vi "poly_notify_by_name_multi.vi"(8 "error in":errorcluster caption="Error in (no error)", 9 "notifier names":string[](array[string]), 10 "name of caller in":string) -> (0 "error out":errorcluster, 1 "notifier refs out":refnum<vi>[](array[refnum]), 4 "notified?":bool[](array[boolean]))   [LabVIEW 2015]
uses:
  ref_tools/polys/poly_control_ref_from_name_caller_multi.vi
  ref_tools/ref_tools_eco.vi
  ref_tools/polys/poly_ref_tools_eco_plus.vi
  error_tools/error_handler.vi
  ref_tools/polys/poly_control_ref_from_name_multi.vi
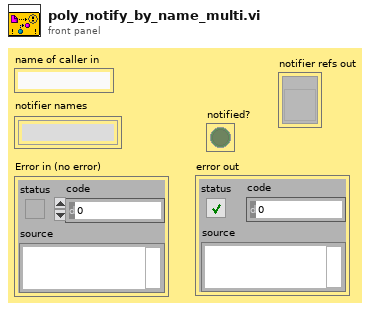
[diagram p1: front panel]
types:
  T1 = typedef "boolean_notifier.ctl" = refnum<notifier>
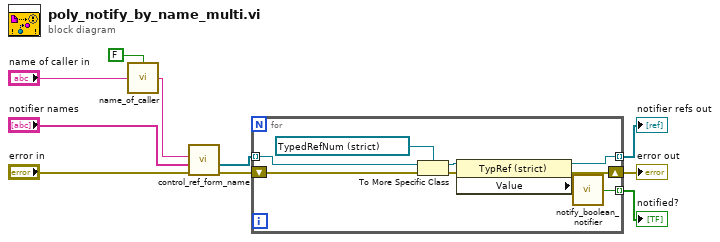
[diagram p0: block diagram]
diagram:
  n1 = call "name_of_caller.vi"("is in inlined vi? (F)"=FALSE, "name of caller in"="name of caller in") -> ("name of caller out"=w6:string)  [unwired: 2 in]
  n2 = call-poly "control_ref_form_name.vi"("error in"="error in", "control names"="notifier names", "name of caller in (your caller)"=w6) -> ("error out"=w8:errorcluster, "control refs"=w10:refnum<vi>[])  [unwired: 6 in, 1 out]
  n3 = for {
    tunnel: w10 -> [w19] mode=indexing
    tunnel: [w12] -> w1 mode=indexing
    tunnel: [w11] -> w2 mode=indexing
    shift-right: [w13] -> w7
    shift-left: w8 -> [w15]
    n4 = To More Specific Class(target class=refnum<vi> refnum ("notifier"), reference=w19, error in=w15) -> (specific class reference=w17:refnum<vi>, error out=w14:errorcluster)
    n5 = property class="TypRef (strict)"(reference=w17, error in=w14) -> (reference out=w12:refnum<vi>, error out=w13:errorcluster, "Value"=w16:T1)
    n6 = call "notify_boolean_notifier.vi"("TF notifier"=w16) -> ("notified?"=w11:bool)  [unwired: 8 in]
  }
  "error out" <- w7
  "notified?" <- w2
  "notifier refs out" <- w1
